vi "2014 State Machine.vi"(0 "Toggle Robot Open/Close":bool, 1 "Left Catapult Solenoid Refnum":T10={"DevStatus"={"status"=FALSE, "code"=0, "source"=""}, "Solenoid Module"=enum."Solenoid Module 1", "Forward Solenoid Channel"=enum."Invalid", "Reverse Solenoid Channel"=enum."Invalid"}, 2 "Intake Solenoid Refnum":T10={"DevStatus"={"status"=FALSE, "code"=0, "source"=""}, "Solenoid Module"=enum."Solenoid Module 1", "Forward Solenoid Channel"=enum."Invalid", "Reverse Solenoid Channel"=enum."Invalid"}, 3 "Intake Motor Refnum":T4={"DeviceStatus"={"status"=FALSE, "code"=0, "source"=""}, "Type"=enum."PWM", "PWM"={"Digital Module"=enum."Digital Module 1", "PWM Channel"=enum."Invalid", "DeadBand"={"Name"="", "maxPositivePwm"=0, "minPositivePwm"=0, "centerPwm"=0, "maxNegativePwm"=0, "minNegativePwm"=0, "angularRange"=0}}, "CAN"={"Device Number"=0, "Control Mode"=enum."Percent VBus", "Semaphore"=refnum, "Max Vout"=12.0}, "Invert"=FALSE, "TransformRef"=refnum, "InvTransformRef"=refnum}, 4 "Ball in launcher":bool, 5 "Shoot Over Truss":bool, 7 "Pass":bool, 9 "Shoot for the Goal":bool, 11 "Intake Load":bool, 12 "Hall Effect Catapult":T1, 13 "Right Catapult Solenoid Refnum":T10={"DevStatus"={"status"=FALSE, "code"=0, "source"=""}, "Solenoid Module"=enum."Solenoid Module 1", "Forward Solenoid Channel"=enum."Invalid", "Reverse Solenoid Channel"=enum."Invalid"}, 14 "Stabilizer Refnum":T10={"DevStatus"={"status"=FALSE, "code"=0, "source"=""}, "Solenoid Module"=enum."Solenoid Module 1", "Forward Solenoid Channel"=enum."Invalid", "Reverse Solenoid Channel"=enum."Invalid"}, 15 "Ball in intake":bool) -> ()   [LabVIEW 2013]
uses:
  <vilib>/Rock Robotics/WPI/Solenoid/WPI_SolenoidDevRef.ctl
  <vilib>/Rock Robotics/SystemInterfaces/Typedef/FPGA_TypedefSolenoidModule.ctl
  <vilib>/Rock Robotics/WPI/Solenoid/WPI_SolenoidChannel.ctl
  <vilib>/Rock Robotics/WPI/MotorControl/WPI_MotorControlDeviceRef.ctl
  <vilib>/Rock Robotics/SystemInterfaces/Typedef/FPGA_TypedefDigitalModule.ctl
  <vilib>/Rock Robotics/SystemInterfaces/DIO/FPGA_DIOPWMChannel.ctl
  <vilib>/Rock Robotics/WPI/PWM/WPI_PWMDeadband.ctl
  <vilib>/Rock Robotics/WPI/CAN/Jaguar/SubVIs/WPI_CANJaguar_ControlMode.ctl
  <vilib>/Rock Robotics/WPI/PWM/WPI_PWMTransform_ConPane.ctl
  <vilib>/Rock Robotics/WPI/DigitalInput/WPI_DigitalInputDevRef.ctl
  <vilib>/Rock Robotics/SystemInterfaces/DIO/FPGA_DIOChannel.ctl
  <vilib>/Rock Robotics/WPI/Solenoid/WPI_SolenoidValue.ctl
  <vilib>/Rock Robotics/WPI/Solenoid/WPI_SolenoidSetEnum.vi
  <vilib>/Rock Robotics/WPI/Solenoid/WPI_SolenoidGetEnum.vi
  <vilib>/Rock Robotics/WPI/Solenoid/Deprecated/WPI_SolenoidGetBool.vi
panel:
  in  "Shooter \nDelay Truss (ms)":dbl
  in  "Intake\nDelay Truss (ms)":dbl
  in  "Shooter \nDelay (ms)":dbl
  in  "Intake\nDelay (ms)":dbl
  in  "Intake Motor Control":dbl(knob) scale=0.0..1.0
  in  "Pass Motor Control":dbl(knob)=-1.0
  out "Current State":T13(ring)
  # "Light switches are auto, vertical switches  are button"
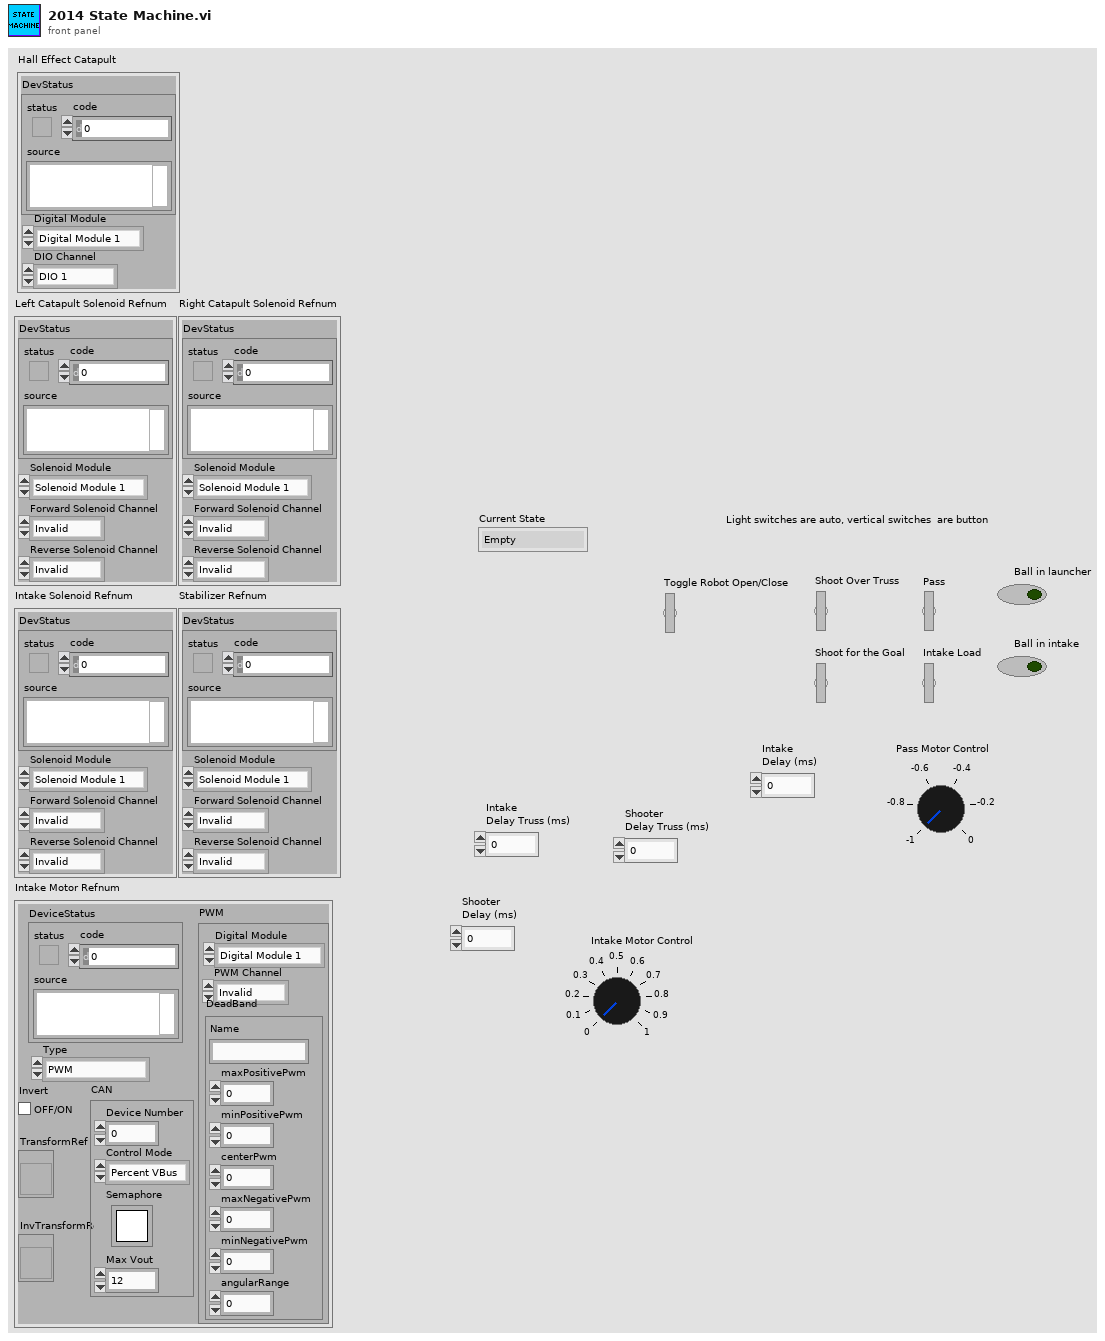
[diagram p1: front panel]
types:
  T1 = typedef "WPI_DigitalInputDevRef.ctl" = cluster{"DevStatus":errorcluster, "DIO Channel":T2, "Digital Module":T3}
  T2 = typedef "FPGA_DIOChannel.ctl" = enum8{"DIO 1", "DIO 2", "DIO 3", "DIO 4", "DIO 5", "DIO 6", "DIO 7", "DIO 8", "DIO 9", "DIO 10", "DIO 11", "DIO 12", "DIO 13", "DIO 14", "Invalid"}
  T3 = typedef "FPGA_TypedefDigitalModule.ctl" = enum16{"Digital Module 1", "Digital Module 2"}
  T4 = typedef "WPI_MotorControlDeviceRef.ctl" = cluster{"DeviceStatus":errorcluster, "Type":enum16{"PWM", "CAN"}, "PWM":cluster{"Digital Module":T3, "PWM Channel":T5, "DeadBand":T6}, "CAN":cluster{"Device Number":u8, "Control Mode":T7, "Semaphore":T8, "Max Vout":dbl}, "Invert":bool, "TransformRef":T9, "InvTransformRef":T9}
  T5 = typedef "FPGA_DIOPWMChannel.ctl" = enum8{"PWM 1", "PWM 2", "PWM 3", "PWM 4", "PWM 5", "PWM 6", "PWM 7", "PWM 8", "PWM 9", "PWM 10", "Invalid"}
  T6 = typedef "WPI_PWMDeadband.ctl" = cluster{"Name":string, "maxPositivePwm":i32, "minPositivePwm":i32, "centerPwm":i32, "maxNegativePwm":i32, "minNegativePwm":i32, "angularRange":u16}
  T7 = typedef "WPI_CANJaguar_ControlMode.ctl" = enum8{"Percent VBus", "Current", "Speed", "Position", "Voltage"}
  T8 = typedef "Semaphore RefNum" = refnum<k1>
  T9 = typedef "WPI_PWMTransform_ConPane.ctl" = refnum<vi>
  T10 = typedef "WPI_SolenoidDevRef.ctl" = cluster{"DevStatus":errorcluster, "Solenoid Module":T11, "Forward Solenoid Channel":T12, "Reverse Solenoid Channel":T12}
  T11 = typedef "FPGA_TypedefSolenoidModule.ctl" = enum16{"Solenoid Module 1", "Solenoid Module 2"}
  T12 = typedef "WPI_SolenoidChannel.ctl" = enum8{"Solenoid 1", "Solenoid 2", "Solenoid 3", "Solenoid 4", "Solenoid 5", "Solenoid 6", "Solenoid 7", "Solenoid 8", "Invalid"}
  T13 = enum16{"Empty", "Catching", "Ball in Intake", "Loaded", "Fire Goal", "Fire Truss"}
  T14 = typedef "WPI_SolenoidValue.ctl" = enum16{"Off", "On", "Forward", "Reverse"}
  T15 = enum16{"Goal Shot", "Truss Shot", "Salveon Says Nadda"}
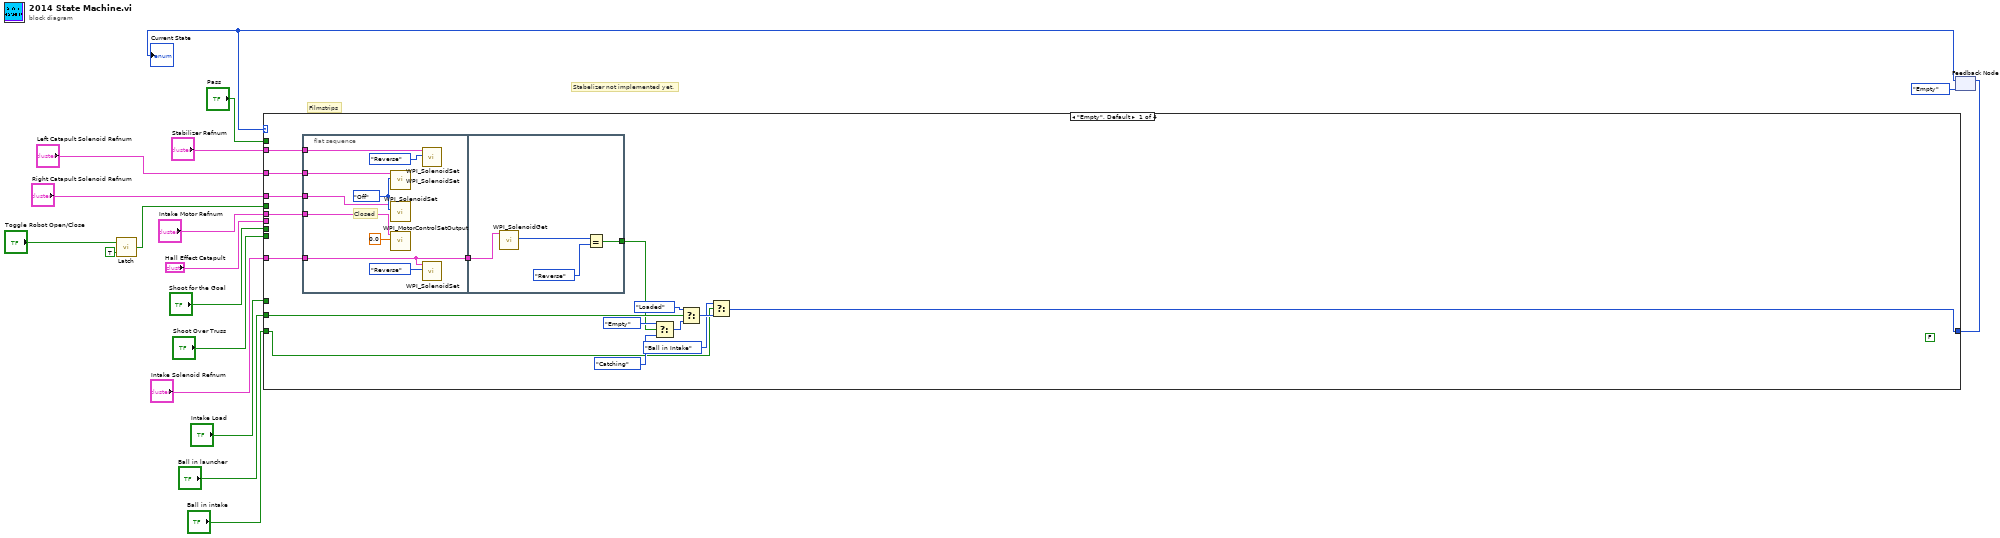
[diagram p0: block diagram]
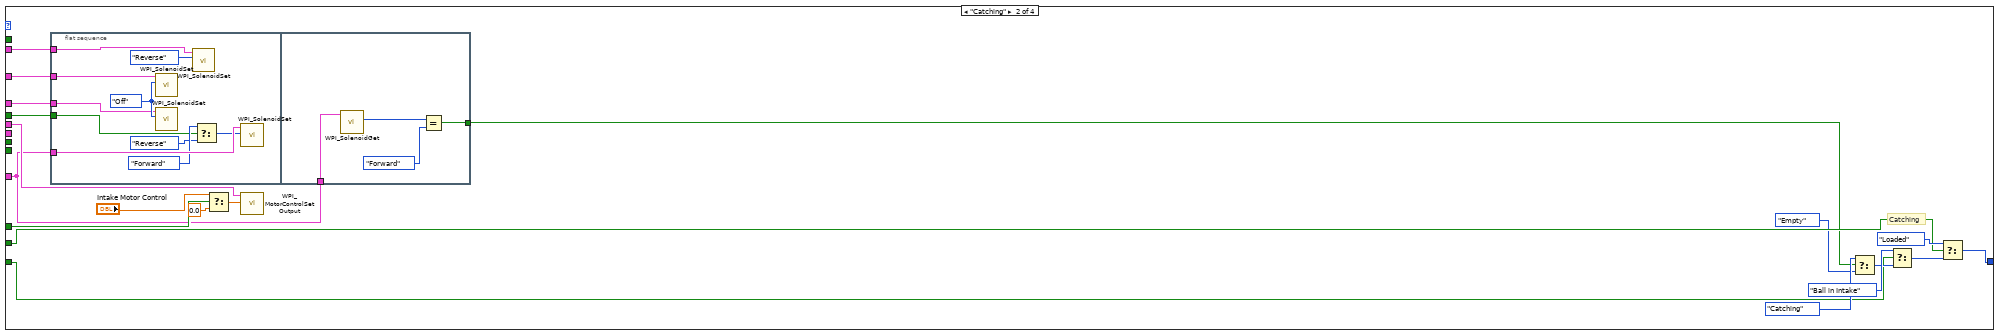
[diagram p2: hidden frame]
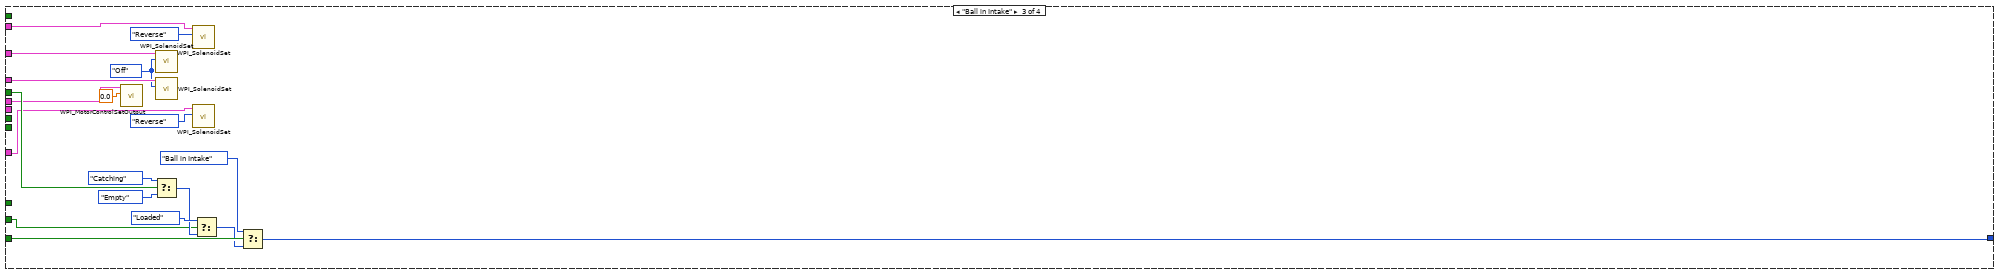
[diagram p3: hidden frame]
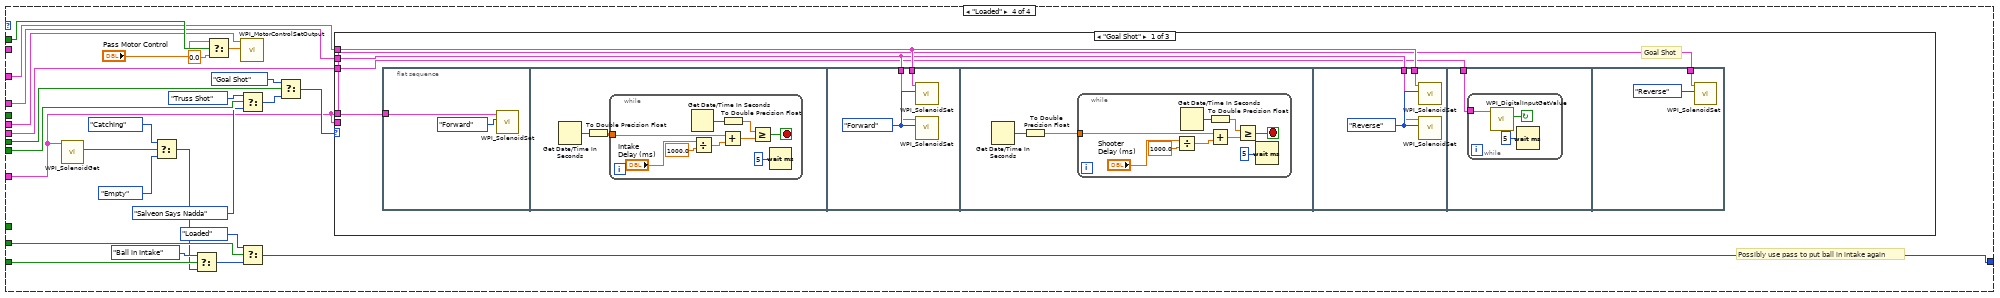
[diagram p4: hidden frame]
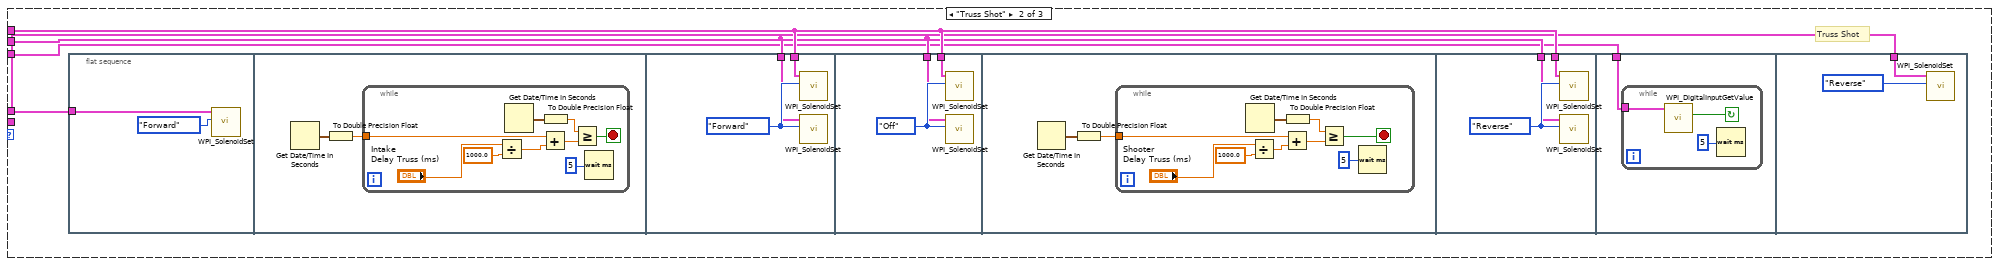
[diagram p5: hidden frame]
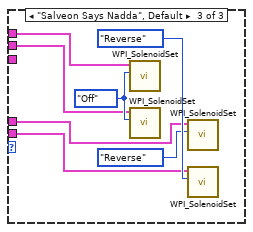
[diagram p6: hidden frame]
diagram:
  # "Stabelizer not implemented yet."
  # "Filmstrips"
  n1 = call "Latch.vi"("Edge"=TRUE, "In"="Toggle Robot Open/Close") -> ("Out"=w7:bool)
  n2 = feedback #1(T13."Empty" ("Robot States")) -> (w10:T13)
  "Current State" <- w10
  n3 = case shown="\"Empty\", Default" w10 {
    tunnel: [w27 w63 w92 w117] -> w11
    tunnel: "Shoot Over Truss" -> [_ _ _ w108]
    tunnel: "Shoot for the Goal" -> [_ _ _ w110]
    tunnel: "Ball in launcher" -> [w31 w61 w91 w122]
    tunnel: "Ball in intake" -> [w26 w60 w100 w120]
    tunnel: "Pass" -> [_ _ _ w116]
    tunnel: "Intake Load" -> [_ w58 _ _]
    tunnel: w7 -> [_ w52 w95 _]
    tunnel: "Intake Motor Refnum" -> [w25 w56 w90 w114]
    tunnel: "Intake Solenoid Refnum" -> [w24 w48 w89 w101]
    tunnel: "Stabilizer Refnum" -> [w23 w51 w88 _]
    tunnel: "Left Catapult Solenoid Refnum" -> [w22 w54 w87 w105]
    tunnel: "Right Catapult Solenoid Refnum" -> [w21 w55 w86 w104]
    tunnel: "Hall Effect Catapult" -> [_ _ _ w103]
    frame "Empty", Default {
      (unwired) FALSE
      n4 = flat-sequence {
        tunnel: w25 -> [w43]
        tunnel: w24 -> [w36]
        tunnel: w23 -> [w40]
        tunnel: w22 -> [w38]
        tunnel: w21 -> [w37]
        tunnel: [w36] -> w20
        tunnel: w20 -> [w47]
        tunnel: [w44] -> w19
        frame #0 {
          w39 = WPI_SolenoidValue."Off" ("Value")
          # "Closed"
          n5 = call-poly <vilib>:"WPI_SolenoidSet.vi"("Value"=w39, "SolenoidDevRef"=w38) -> ()  [unwired: 8 in, 2 out]
          n6 = call-poly <vilib>:"WPI_SolenoidSet.vi"("Value"=w39, "SolenoidDevRef"=w37) -> ()  [unwired: 8 in, 2 out]
          n7 = call <vilib>:"WPI_MotorControlSetOutput.vi"("Output"=0.0, "MotorControlDevRef"=w43) -> ()  [unwired: 7 in, 3 out]
          n8 = call-poly <vilib>:"WPI_SolenoidSet.vi"("Value"=WPI_SolenoidValue."Reverse", "SolenoidDevRef"=w40) -> ()  [unwired: 8 in, 2 out]
          n9 = call-poly <vilib>:"WPI_SolenoidSet.vi"("Value"=WPI_SolenoidValue."Reverse", "SolenoidDevRef"=w36) -> ()  [unwired: 8 in, 2 out]
        }
        frame #1 {
          n10 = call-poly <vilib>:"WPI_SolenoidGet.vi"("SolenoidDevRef"=w47) -> ("Value"=w46:T14)  [unwired: 8 in, 2 out]
          n11 = Equal?(x=w46, y=WPI_SolenoidValue."Reverse") -> (x = y?=w44:bool)
        }
      }
      n12 = Select(t=T13."Empty" ("Robot States"), s=w19, f=T13."Catching" ("Robot States")) -> (s? t:f=w32:T13)
      n13 = Select(t=T13."Loaded" ("Robot States"), s=w31, f=w32) -> (s? t:f=w29:T13)
      n14 = Select(t=T13."Ball in Intake" ("Robot States"), s=w26, f=w29) -> (s? t:f=w27:T13)
    }
    frame "Catching" {
      # "Catching"
      n15 = flat-sequence {
        tunnel: w51 -> [w76]
        tunnel: w55 -> [w74]
        tunnel: w54 -> [w73]
        tunnel: w48 -> [w72]
        tunnel: w52 -> [w68]
        tunnel: [w79] -> w49
        tunnel: w48 -> [w78]
        frame #0 {
          w75 = WPI_SolenoidValue."Off" ("Value")
          n16 = call-poly <vilib>:"WPI_SolenoidSet.vi"("Value"=w75, "SolenoidDevRef"=w73) -> ()  [unwired: 8 in, 2 out]
          n17 = call-poly <vilib>:"WPI_SolenoidSet.vi"("Value"=w75, "SolenoidDevRef"=w74) -> ()  [unwired: 8 in, 2 out]
          n18 = call-poly <vilib>:"WPI_SolenoidSet.vi"("Value"=WPI_SolenoidValue."Reverse", "SolenoidDevRef"=w76) -> ()  [unwired: 8 in, 2 out]
          n19 = Select(t=WPI_SolenoidValue."Forward" ("Value"), s=w68, f=WPI_SolenoidValue."Reverse") -> (s? t:f=w70:T14)
          n20 = call-poly <vilib>:"WPI_SolenoidSet.vi"("Value"=w70, "SolenoidDevRef"=w72) -> ()  [unwired: 8 in, 2 out]
        }
        frame #1 {
          n21 = call-poly <vilib>:"WPI_SolenoidGet.vi"("SolenoidDevRef"=w78) -> ("Value"=w81:T14)  [unwired: 8 in, 2 out]
          n22 = Equal?(x=w81, y=WPI_SolenoidValue."Forward") -> (x = y?=w79:bool)
        }
      }
      n23 = Select(t="Intake Motor Control", s=w58, f=0.0) -> (s? t:f=w57:dbl)
      n24 = call <vilib>:"WPI_MotorControlSetOutput.vi"("Output"=w57, "MotorControlDevRef"=w56) -> ()  [unwired: 7 in, 3 out]
      n25 = Select(t=T13."Catching" ("Robot States"), s=w49, f=T13."Empty") -> (s? t:f=w62:T13)
      n26 = Select(t=T13."Ball in Intake" ("Robot States"), s=w60, f=w62) -> (s? t:f=w67:T13)
      n27 = Select(t=T13."Loaded" ("Robot States"), s=w61, f=w67) -> (s? t:f=w63:T13)
    }
    frame "Ball in Intake" {
      w83 = WPI_SolenoidValue."Off" ("Value")
      n28 = call <vilib>:"WPI_MotorControlSetOutput.vi"("Output"=0.0 ("f"), "MotorControlDevRef"=w90) -> ()  [unwired: 7 in, 3 out]
      n29 = call-poly <vilib>:"WPI_SolenoidSet.vi"("Value"=w83, "SolenoidDevRef"=w87) -> ()  [unwired: 8 in, 2 out]
      n30 = call-poly <vilib>:"WPI_SolenoidSet.vi"("Value"=w83, "SolenoidDevRef"=w86) -> ()  [unwired: 8 in, 2 out]
      n31 = Select(t=T13."Catching" ("Robot States"), s=w95, f=T13."Empty" ("Robot States")) -> (s? t:f=w96:T13)
      n32 = call-poly <vilib>:"WPI_SolenoidSet.vi"("Value"=WPI_SolenoidValue."Reverse", "SolenoidDevRef"=w88) -> ()  [unwired: 8 in, 2 out]
      n33 = call-poly <vilib>:"WPI_SolenoidSet.vi"("Value"=WPI_SolenoidValue."Reverse", "SolenoidDevRef"=w89) -> ()  [unwired: 8 in, 2 out]
      n34 = Select(t=T13."Loaded" ("Robot States"), s=w91, f=w96) -> (s? t:f=w98:T13)
      n35 = Select(t=T13."Ball in Intake" ("Robot States"), s=w100, f=w98) -> (s? t:f=w92:T13)
    }
    frame "Loaded" {
      # "Possibly use pass to put ball in intake again"
      n36 = call-poly <vilib>:"WPI_SolenoidGet.vi"("SolenoidDevRef"=w101) -> ("Value"=w102:bool)  [unwired: 8 in, 2 out]
      n37 = Select(t=T13."Catching" ("Robot States"), s=w102, f=T13."Empty" ("Robot States")) -> (s? t:f=w118:T13)
      n38 = Select(t=T13."Ball in Intake" ("Robot States"), s=w120, f=w118) -> (s? t:f=w121:T13)
      n39 = Select(t="Pass Motor Control", s=w116, f=0.0) -> (s? t:f=w115:dbl)
      n40 = call <vilib>:"WPI_MotorControlSetOutput.vi"("Output"=w115, "MotorControlDevRef"=w114) -> ()  [unwired: 7 in, 3 out]
      n41 = Select(t=T15."Truss Shot" ("Enum"), s=w108, f=T15."Salveon Says Nadda" ("Enum")) -> (s? t:f=w112:T15)
      n42 = Select(t=T13."Loaded" ("Robot States"), s=w122, f=w121) -> (s? t:f=w117:T13)
      n43 = Select(t=T15."Goal Shot" ("Enum"), s=w110, f=w112) -> (s? t:f=w111:T15)
      n44 = case shown="\"Goal Shot\"" w111 {
        tunnel: w101 -> [_ _ w215]
        tunnel: w105 -> [w130 w170 w212]
        tunnel: w104 -> [w129 w169 w211]
        tunnel: w101 -> [w127 w167 w210]
        tunnel: w103 -> [w128 w168 _]
        frame "Goal Shot" {
          # "Goal Shot"
          n45 = flat-sequence {
            tunnel: w127 -> [w132]
            tunnel: w130 -> [w145]
            tunnel: w129 -> [w144]
            tunnel: w130 -> [w159]
            tunnel: w129 -> [w158]
            tunnel: w128 -> [w161]
            tunnel: w127 -> [w165]
            frame #0 {
              n46 = call-poly <vilib>:"WPI_SolenoidSet.vi"("Value"=WPI_SolenoidValue."Forward", "SolenoidDevRef"=w132) -> ()  [unwired: 8 in, 2 out]
            }
            frame #1 {
              n47 = Get Date/Time In Seconds() -> (seconds since 1Jan1904=w134:timestamp)
              n48 = To Double Precision Float(number=w134) -> (double precision float=w133:dbl)
              n49 = while {
                tunnel: w133 -> [w137]
                stop <- w141 stop-if-true
                n50 = Get Date/Time In Seconds() -> (seconds since 1Jan1904=w143:timestamp)
                n51 = Divide(x="Intake\nDelay (ms)", y=1000.0) -> (x/y=w138:dbl)
                n52 = Add(x=w137, y=w138) -> (x+y=w136:dbl)
                n53 = To Double Precision Float(number=w143) -> (double precision float=w142:dbl)
                n54 = Greater Or Equal?(x=w142, y=w136) -> (x >= y?=w141:bool)
                n55 = Wait (ms)(milliseconds to wait=u32 5) -> ()  [unwired: 1 out]
              }
            }
            frame #2 {
              w146 = WPI_SolenoidValue."Forward" ("Value")
              n56 = call-poly <vilib>:"WPI_SolenoidSet.vi"("Value"=w146, "SolenoidDevRef"=w145) -> ()  [unwired: 8 in, 2 out]
              n57 = call-poly <vilib>:"WPI_SolenoidSet.vi"("Value"=w146, "SolenoidDevRef"=w144) -> ()  [unwired: 8 in, 2 out]
            }
            frame #3 {
              n58 = Get Date/Time In Seconds() -> (seconds since 1Jan1904=w148:timestamp)
              n59 = To Double Precision Float(number=w148) -> (double precision float=w147:dbl)
              n60 = while {
                tunnel: w147 -> [w152]
                stop <- w155 stop-if-true
                n61 = Divide(x="Shooter \nDelay (ms)", y=1000.0) -> (x/y=w151:dbl)
                n62 = Get Date/Time In Seconds() -> (seconds since 1Jan1904=w157:timestamp)
                n63 = Add(x=w152, y=w151) -> (x+y=w150:dbl)
                n64 = To Double Precision Float(number=w157) -> (double precision float=w156:dbl)
                n65 = Greater Or Equal?(x=w156, y=w150) -> (x >= y?=w155:bool)
                n66 = Wait (ms)(milliseconds to wait=u32 5) -> ()  [unwired: 1 out]
              }
            }
            frame #4 {
              w160 = WPI_SolenoidValue."Reverse" ("Value")
              n67 = call-poly <vilib>:"WPI_SolenoidSet.vi"("Value"=w160, "SolenoidDevRef"=w159) -> ()  [unwired: 8 in, 2 out]
              n68 = call-poly <vilib>:"WPI_SolenoidSet.vi"("Value"=w160, "SolenoidDevRef"=w158) -> ()  [unwired: 8 in, 2 out]
            }
            frame #5 {
              n69 = while {
                tunnel: w161 -> [w164]
                stop <- w163 continue-if-true
                n70 = call <vilib>:"WPI_DigitalInputGetValue.vi"("DigitalInputDevRef"=w164) -> ("Value"=w163:bool)  [unwired: 8 in, 2 out]
                n71 = Wait (ms)(milliseconds to wait=u32 5) -> ()  [unwired: 1 out]
              }
            }
            frame #6 {
              n72 = call-poly <vilib>:"WPI_SolenoidSet.vi"("Value"=WPI_SolenoidValue."Reverse", "SolenoidDevRef"=w165) -> ()  [unwired: 8 in, 2 out]
            }
          }
        }
        frame "Truss Shot" {
          # "Truss Shot"
          n73 = flat-sequence {
            tunnel: w167 -> [w171]
            tunnel: w170 -> [w185]
            tunnel: w169 -> [w184]
            tunnel: w170 -> [w188]
            tunnel: w169 -> [w187]
            tunnel: w170 -> [w202]
            tunnel: w169 -> [w201]
            tunnel: w168 -> [w204]
            tunnel: w167 -> [w208]
            frame #0 {
              n74 = call-poly <vilib>:"WPI_SolenoidSet.vi"("Value"=WPI_SolenoidValue."Forward", "SolenoidDevRef"=w171) -> ()  [unwired: 8 in, 2 out]
            }
            frame #1 {
              n75 = Get Date/Time In Seconds() -> (seconds since 1Jan1904=w174:timestamp)
              n76 = To Double Precision Float(number=w174) -> (double precision float=w173:dbl)
              n77 = while {
                tunnel: w173 -> [w177]
                stop <- w181 stop-if-true
                n78 = Divide(x="Intake\nDelay Truss (ms)", y=1000.0) -> (x/y=w178:dbl)
                n79 = Get Date/Time In Seconds() -> (seconds since 1Jan1904=w183:timestamp)
                n80 = Add(x=w177, y=w178) -> (x+y=w176:dbl)
                n81 = To Double Precision Float(number=w183) -> (double precision float=w182:dbl)
                n82 = Greater Or Equal?(x=w182, y=w176) -> (x >= y?=w181:bool)
                n83 = Wait (ms)(milliseconds to wait=u32 5) -> ()  [unwired: 1 out]
              }
            }
            frame #2 {
              w186 = WPI_SolenoidValue."Forward" ("Value")
              n84 = call-poly <vilib>:"WPI_SolenoidSet.vi"("Value"=w186, "SolenoidDevRef"=w185) -> ()  [unwired: 8 in, 2 out]
              n85 = call-poly <vilib>:"WPI_SolenoidSet.vi"("Value"=w186, "SolenoidDevRef"=w184) -> ()  [unwired: 8 in, 2 out]
            }
            frame #3 {
              w189 = WPI_SolenoidValue."Off" ("Value")
              n86 = call-poly <vilib>:"WPI_SolenoidSet.vi"("Value"=w189, "SolenoidDevRef"=w188) -> ()  [unwired: 8 in, 2 out]
              n87 = call-poly <vilib>:"WPI_SolenoidSet.vi"("Value"=w189, "SolenoidDevRef"=w187) -> ()  [unwired: 8 in, 2 out]
            }
            frame #4 {
              n88 = Get Date/Time In Seconds() -> (seconds since 1Jan1904=w191:timestamp)
              n89 = To Double Precision Float(number=w191) -> (double precision float=w190:dbl)
              n90 = while {
                tunnel: w190 -> [w195]
                stop <- w198 stop-if-true
                n91 = Get Date/Time In Seconds() -> (seconds since 1Jan1904=w200:timestamp)
                n92 = Divide(x="Shooter \nDelay Truss (ms)", y=1000.0) -> (x/y=w194:dbl)
                n93 = Add(x=w195, y=w194) -> (x+y=w193:dbl)
                n94 = To Double Precision Float(number=w200) -> (double precision float=w199:dbl)
                n95 = Greater Or Equal?(x=w199, y=w193) -> (x >= y?=w198:bool)
                n96 = Wait (ms)(milliseconds to wait=u32 5) -> ()  [unwired: 1 out]
              }
            }
            frame #5 {
              w203 = WPI_SolenoidValue."Reverse" ("Value")
              n97 = call-poly <vilib>:"WPI_SolenoidSet.vi"("Value"=w203, "SolenoidDevRef"=w202) -> ()  [unwired: 8 in, 2 out]
              n98 = call-poly <vilib>:"WPI_SolenoidSet.vi"("Value"=w203, "SolenoidDevRef"=w201) -> ()  [unwired: 8 in, 2 out]
            }
            frame #6 {
              n99 = while {
                tunnel: w204 -> [w206]
                stop <- w207 continue-if-true
                n100 = call <vilib>:"WPI_DigitalInputGetValue.vi"("DigitalInputDevRef"=w206) -> ("Value"=w207:bool)  [unwired: 8 in, 2 out]
                n101 = Wait (ms)(milliseconds to wait=u32 5) -> ()  [unwired: 1 out]
              }
            }
            frame #7 {
              n102 = call-poly <vilib>:"WPI_SolenoidSet.vi"("Value"=WPI_SolenoidValue."Reverse", "SolenoidDevRef"=w208) -> ()  [unwired: 8 in, 2 out]
            }
          }
        }
        frame "Salveon Says Nadda", Default {
          w213 = WPI_SolenoidValue."Off" ("Value")
          n103 = call-poly <vilib>:"WPI_SolenoidSet.vi"("Value"=w213, "SolenoidDevRef"=w212) -> ()  [unwired: 8 in, 2 out]
          n104 = call-poly <vilib>:"WPI_SolenoidSet.vi"("Value"=w213, "SolenoidDevRef"=w211) -> ()  [unwired: 8 in, 2 out]
          n105 = call-poly <vilib>:"WPI_SolenoidSet.vi"("Value"=WPI_SolenoidValue."Reverse", "SolenoidDevRef"=w210) -> ()  [unwired: 8 in, 2 out]
          n106 = call-poly <vilib>:"WPI_SolenoidSet.vi"("Value"=WPI_SolenoidValue."Reverse", "SolenoidDevRef"=w215) -> ()  [unwired: 8 in, 2 out]
        }
      }
    }
  }
  n107 = feedback-in #1(w11) -> ()
